vi "Super Market Billing System Add Products.vi"() -> ()   [LabVIEW 2021]
panel:
  in  "Quantity":dbl=1.0 min=1.0 max=10.0
  in  "Quantity":dbl=1.0 min=1.0 max=10.0
  in  "Quantity":dbl=1.0 min=1.0 max=10.0
  in  "Quantity":dbl=1.0 min=1.0 max=10.0
  in  "Quantity":dbl=1.0 min=1.0 max=10.0
  in  "Quantity":dbl=1.0 min=1.0 max=10.0
  in  "Quantity":dbl=1.0 min=1.0 max=10.0
  in  "Quantity":dbl=1.0 min=1.0 max=10.0
  in  "Quantity":dbl=1.0 min=1.0 max=10.0
  in  "Quantity":dbl=1.0 min=1.0 max=10.0
  out "Price":dbl
  out "Price":dbl
  out "Price":dbl
  out "Price":dbl
  out "Price":dbl
  out "Price":dbl
  out "Price":dbl
  out "Price":dbl
  out "Price":dbl
  out "Price":dbl
  in  "Turmeric Powder 50g":bool
  in  "Curry Powder 100g":bool
  in  "Cilli Powder 100g":bool
  in  "Coconut Oil 1L":bool
  in  "Salt 400g":bool
  in  "Dal 1kg":bool
  in  "Tea 100g":bool
  in  "Sugar 1kg":bool
  in  "Milk Powder 1kg":bool
  in  "Rice 5kg":bool
  out "Bill":dbl
  # "Product List"
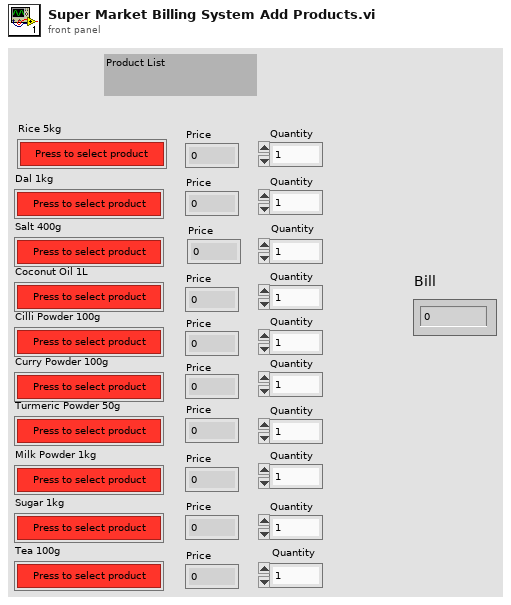
[diagram p1: front panel]
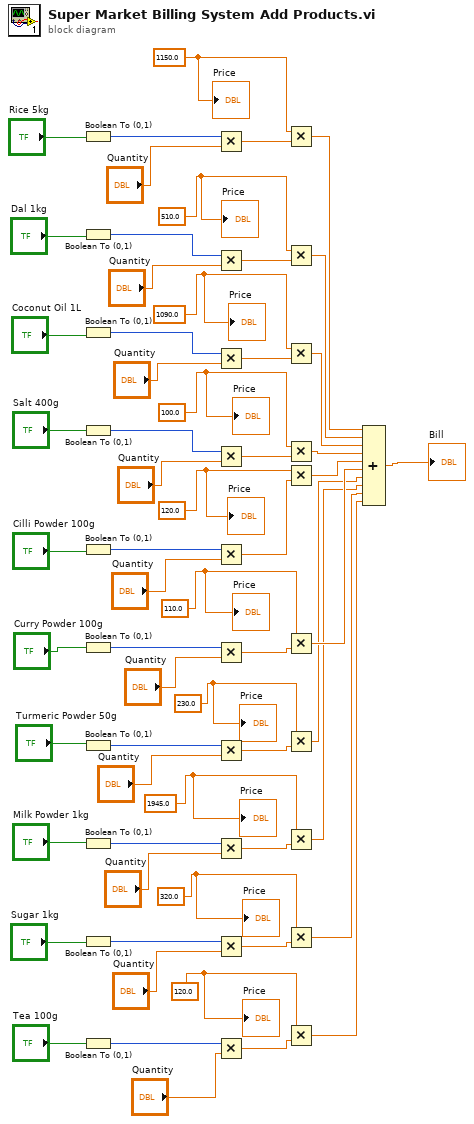
[diagram p0: block diagram]
diagram:
  w16 = 120.0 ("price")
  w17 = 100.0 ("price")
  w18 = 1090.0 ("price")
  w19 = 510.0 ("price")
  w20 = 1150.0 ("price")
  w11 = 120.0 ("price")
  w12 = 320.0 ("price")
  w13 = 1945.0 ("price")
  w14 = 230.0 ("price")
  w15 = 110.0 ("price")
  n1 = Boolean To (0,1)(Boolean="Rice 5kg") -> (0, 1=w37:i16)
  n2 = Boolean To (0,1)(Boolean="Dal 1kg") -> (0, 1=w40:i16)
  n3 = Boolean To (0,1)(Boolean="Coconut Oil 1L") -> (0, 1=w41:i16)
  n4 = Boolean To (0,1)(Boolean="Salt 400g") -> (0, 1=w44:i16)
  n5 = Boolean To (0,1)(Boolean="Cilli Powder 100g") -> (0, 1=w45:i16)
  n6 = Boolean To (0,1)(Boolean="Curry Powder 100g") -> (0, 1=w52:i16)
  n7 = Boolean To (0,1)(Boolean="Turmeric Powder 50g") -> (0, 1=w55:i16)
  n8 = Boolean To (0,1)(Boolean="Milk Powder 1kg") -> (0, 1=w56:i16)
  n9 = Boolean To (0,1)(Boolean="Sugar 1kg") -> (0, 1=w59:i16)
  n10 = Boolean To (0,1)(Boolean="Tea 100g") -> (0, 1=w60:i16)
  n11 = Multiply(x=w37, y="Quantity") -> (x*y=w38:dbl)
  n12 = Multiply(x=w40, y="Quantity") -> (x*y=w39:dbl)
  n13 = Multiply(x=w41, y="Quantity") -> (x*y=w42:dbl)
  n14 = Multiply(x=w44, y="Quantity") -> (x*y=w43:dbl)
  n15 = Multiply(x=w45, y="Quantity") -> (x*y=w46:dbl)
  n16 = Multiply(x=w52, y="Quantity") -> (x*y=w53:dbl)
  n17 = Multiply(x=w55, y="Quantity") -> (x*y=w54:dbl)
  n18 = Multiply(x=w56, y="Quantity") -> (x*y=w57:dbl)
  n19 = Multiply(x=w59, y="Quantity") -> (x*y=w58:dbl)
  n20 = Multiply(x=w60, y="Quantity") -> (x*y=w61:dbl)
  n21 = Multiply(x=w20, y=w38) -> (x*y=w47:dbl)
  n22 = Multiply(x=w19, y=w39) -> (x*y=w48:dbl)
  n23 = Multiply(x=w18, y=w42) -> (x*y=w49:dbl)
  n24 = Multiply(x=w17, y=w43) -> (x*y=w50:dbl)
  n25 = Multiply(x=w16, y=w46) -> (x*y=w51:dbl)
  n26 = Multiply(x=w15, y=w53) -> (x*y=w35:dbl)
  n27 = Multiply(x=w14, y=w54) -> (x*y=w34:dbl)
  n28 = Multiply(x=w13, y=w57) -> (x*y=w33:dbl)
  n29 = Multiply(x=w12, y=w58) -> (x*y=w32:dbl)
  n30 = Multiply(x=w11, y=w61) -> (x*y=w31:dbl)
  n31 = Compound Arithmetic op=ADD(w47, w48, w49, w50, w51, w35, w34, w33, w32, w31) -> (→"Bill":dbl)
  "Price" <- w20
  "Price" <- w19
  "Price" <- w18
  "Price" <- w17
  "Price" <- w16
  "Price" <- w15
  "Price" <- w14
  "Price" <- w13
  "Price" <- w12
  "Price" <- w11
